vi "GetSize.vi"(8 "error in (no error)":errorcluster, 11 "reference in":refnum<class "Character.lvclass">) -> (0 "error out":errorcluster, 2 "Dimensions":T1, 3 "reference in":refnum<class "Character.lvclass">)   [LabVIEW 2012, in "Character.lvclass"]
uses:
  Character.lvclass
  Glyph_class/Dimensions.ctl
  Glyph_class/Glyph.lvclass
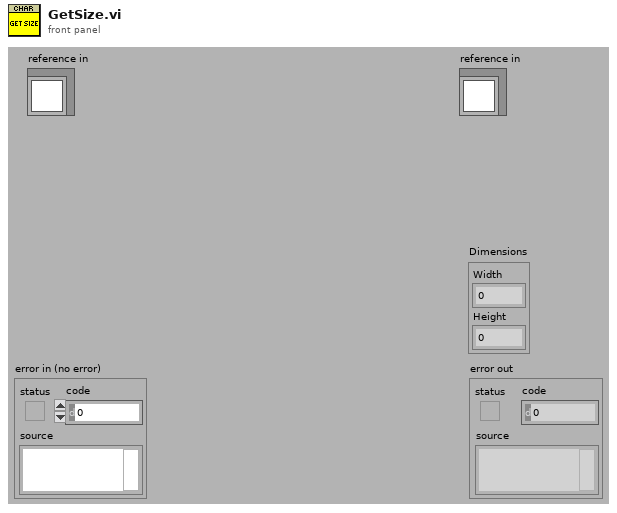
[diagram p1: front panel]
types:
  T1 = typedef "Glyph.lvclass/Dimensions.ctl" = cluster{"Width":i32, "Height":i32}
  T2 = enum16{"User-specified Font", "Application Font", "System Font", "Dialog Font"}
  T3 = typedef "Character.lvclass/ObjectAttributes.ctl" = cluster{"Font":cluster{"Font Name:":string, "Size":i16, "Strikeout?":bool, "Italic?":bool, "Underline?":bool, "Outline?":bool, "Shadow?":bool, "Bold?":bool}, "Color":u32, "Character":string}
  T4 = cluster{"Font Name:":string, "Size":i16, "Strikeout?":bool, "Italic?":bool, "Underline?":bool, "Outline?":bool, "Shadow?":bool, "Bold?":bool}
  T5 = cluster{"left":i16, "top":i16, "right":i16, "bottom":i16}
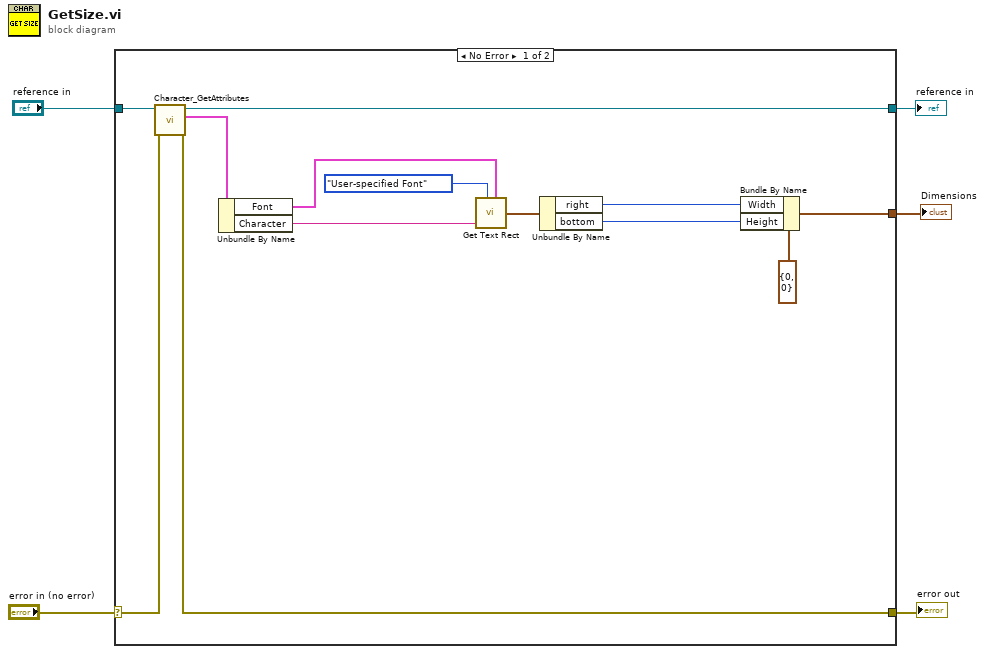
[diagram p0: block diagram]
diagram:
  n1 = case shown="No Error" "error in (no error)" {
    selector: "error in (no error)" -> [w18 w20]
    tunnel: [w16 w20] -> w4
    tunnel: [w14 w19] -> w2
    tunnel: "reference in" -> [w15 w19]
    tunnel: [w6 _] -> w1
    frame No Error {
      n2 = call "Character_GetAttributes.vi"("error in (no error)"=w18, "reference in"=w15) -> ("error out"=w16:errorcluster, "Data"=w17:T3, "reference out"=w14:refnum<class "Character.lvclass">)  [unwired: 6 in, 1 out]
      n3 = Unbundle By Name(w17) -> ("Font"=w12:T4, "Character"=w13:string)
      n4 = call <vilib>:"Get Text Rect.vi"("desired font(Application)"=T2."User-specified Font", "text"=w13, "[user-specified font]"=w12) -> ("rect"=w10:T5)  [unwired: 6 in]
      n5 = Unbundle By Name(w10) -> ("right"=w8:i16, "bottom"=w7:i16)
      n6 = Bundle By Name(cluster=T1 {"Width"=0, "Height"=0} ("Dimensions"), "Width"=w8, "Height"=w7) -> (w6:T1)
    }
    frame Error {
    }
  }
  "error out" <- w4
  "reference in" <- w2
  "Dimensions" <- w1
